vi "PH_ImageStatistician.evt Call Select Data.vi"(0 "i ref in":refnum<vi>, 1 "Stat or Trend":bool, 2 "Data 1":T1 items=["nothing ", "FWHM Major Trace", "FWHM Minor Trace", "Gaussian Fit Order Major Trace", "Gaussian Fit Order Minor Trace", "99% Diameter Major Trace", "99% Diameter Minor Trace", "Theta", "Delta", "Major Diameter", "Minor Diameter", "Azimuth Angle", "Azi Angle rel to Major?", "Ellipticity", "Center of gravity - x", "Center of gravity - y", "Energy"], 3 "Data 2":T1 items=["nothing ", "FWHM Major Trace", "FWHM Minor Trace", "Gaussian Fit Order Major Trace", "Gaussian Fit Order Minor Trace", "99% Diameter Major Trace", "99% Diameter Minor Trace", "Theta", "Delta", "Major Diameter", "Minor Diameter", "Azimuth Angle", "Azi Angle rel to Major?", "Ellipticity", "Center of gravity - x", "Center of gravity - y", "Energy"], 4 "Data 3":T1 items=["nothing ", "FWHM Major Trace", "FWHM Minor Trace", "Gaussian Fit Order Major Trace", "Gaussian Fit Order Minor Trace", "99% Diameter Major Trace", "99% Diameter Minor Trace", "Theta", "Delta", "Major Diameter", "Minor Diameter", "Azimuth Angle", "Azi Angle rel to Major?", "Ellipticity", "Center of gravity - x", "Center of gravity - y", "Energy"], 5 "error in (no error)":errorcluster, 6 "Instance":string="N/A") -> (14 "i ref out":refnum<vi>, 19 "error out":errorcluster)   [LabVIEW 2014, in "PH_ImageStatistician.lvlib"]
doc: "This VI calls a certain ProcCase"
uses:
  PH_ImageStatistician.lvlib
  PH_ImageStatistician.select Data.ctl
  CS_Core/CSSystem/CoreLib/CoreLib.short 2 byte array.vi
  CS_Core/BaseProcess/BaseProcess.lvlib
  CS_Core/CSSystem/CoreLib/CoreLib.lvlib
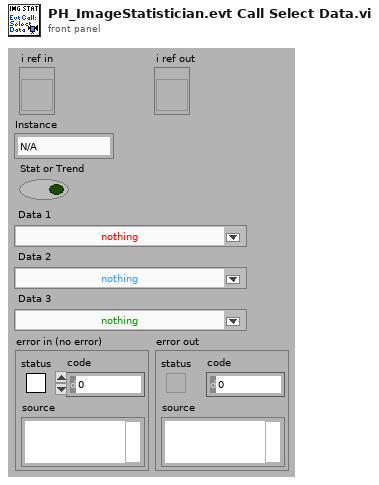
[diagram p1: front panel]
types:
  T1 = typedef "PH_ImageStatistician.lvlib/PH_ImageStatistician.select Data.ctl" = u16
  T2 = typedef "CoreDefs.rawDataType.ctl" = i8[]
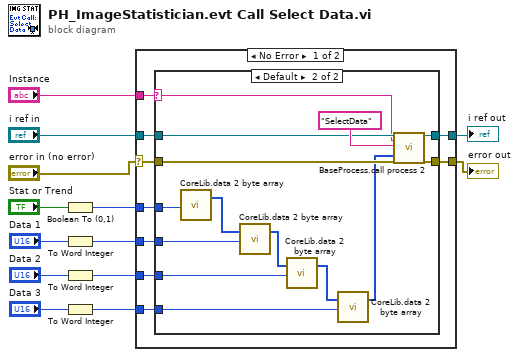
[diagram p0: block diagram]
diagram:
  n1 = Boolean To (0,1)(Boolean="Stat or Trend") -> (0, 1=w7:i16)
  n2 = To Word Integer(number="Data 1") -> (16bit integer=w3:i16)
  n3 = To Word Integer(number="Data 2") -> (16bit integer=w2:i16)
  n4 = To Word Integer(number="Data 3") -> (16bit integer=w1:i16)
  n5 = case shown="No Error" "error in (no error)" {
    selector: "error in (no error)" -> [w18 w39]
    tunnel: [w22 w40] -> w13
    tunnel: [w21 w39] -> w12
    tunnel: "i ref in" -> [w20 w40]
    tunnel: "Instance" -> [w19 _]
    tunnel: w7 -> [w17 _]
    tunnel: w3 -> [w16 _]
    tunnel: w2 -> [w15 _]
    tunnel: w1 -> [w14 _]
    frame No Error {
      n6 = case shown="Default" w19 {
        selector: w19 -> [_ w33]
        tunnel: [w24 w36] -> w22
        tunnel: [w23 w35] -> w21
        tunnel: w20 -> [w24 w34]
        tunnel: w18 -> [w23 w38]
        tunnel: w17 -> [_ w32]
        tunnel: w16 -> [_ w27]
        tunnel: w15 -> [_ w26]
        tunnel: w14 -> [_ w25]
        frame "N/A" {
        }
        frame Default {
          n7 = call-poly "CoreLib.data 2 byte array.vi"("i16"=w32) -> ("byteArray out"=w29:T2)  [unwired: 18 in]
          n8 = call-poly "CoreLib.data 2 byte array.vi"("byteArray"=w29, "i16"=w27) -> ("byteArray out"=w31:T2)  [unwired: 17 in]
          n9 = call-poly "CoreLib.data 2 byte array.vi"("byteArray"=w31, "i16"=w26) -> ("byteArray out"=w30:T2)  [unwired: 17 in]
          n10 = call-poly "CoreLib.data 2 byte array.vi"("byteArray"=w30, "i16"=w25) -> ("byteArray out"=w28:T2)  [unwired: 17 in]
          n11 = call "BaseProcess.call process 2.vi"("i ref in"=w34, "Object"=w33, "Selector"="SelectData", "Data"=w28, "error in (no error)"=w38) -> ("i ref out"=w36:refnum<vi>, "error out"=w35:errorcluster)  [unwired: 13 in]
        }
      }
    }
    frame Error {
    }
  }
  "error out" <- w12
  "i ref out" <- w13
